vi "Update.vi"(8 "error in (no error)":errorcluster, 10 "TimePassed(ms)":i64, 11 "Timer in":refnum<class "Timer.lvclass">) -> (0 "error out":errorcluster, 1 "Triggered?":bool, 2 "UserEvent":T1, 3 "Timer out":refnum<class "Timer.lvclass">)   [LabVIEW 2017, in "TimerEngine.lvlib" / "Timer.lvclass"]
uses:
  Timer.lvclass
  _Typedef/Timer-UserEvent.ctl
  Timer.lvclass/Timer.ctl
  TimerEngine.lvclass
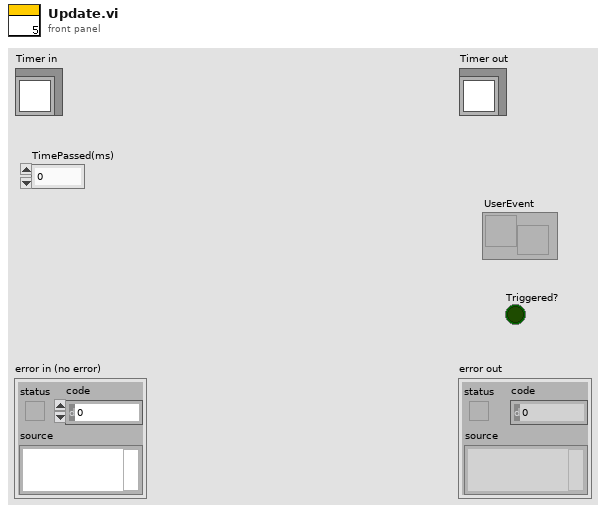
[diagram p1: front panel]
types:
  T1 = typedef "TimerEngine.lvlib/TimerEngine.lvclass/Timer-UserEvent.ctl" = refnum<user-event>
  T2 = typedef "TimerEngine.lvlib/TimerEngine.lvclass/Timer-Userevent.ctl" = refnum<user-event>
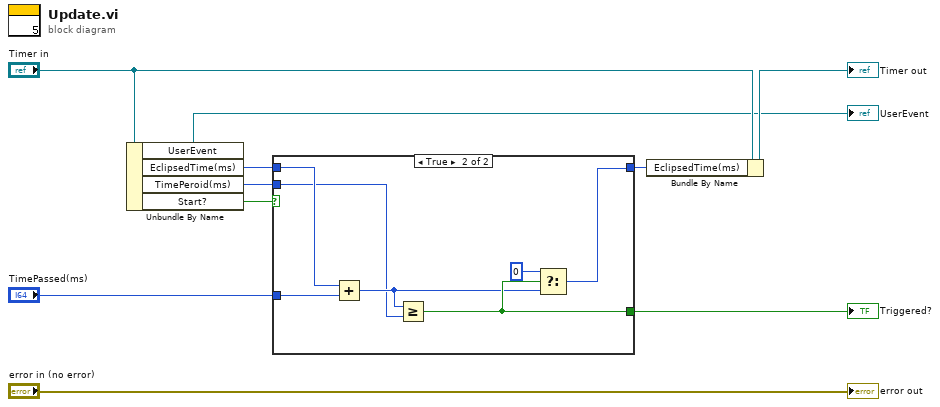
[diagram p0: block diagram]
diagram:
  n1 = Unbundle By Name("Timer in") -> ("UserEvent"=→"UserEvent":T2, "EclipsedTime(ms)"=w9:i64, "TimePeroid(ms)"=w7:i64, "Start?"=w1:bool)
  n2 = case shown="True" w1 {
    tunnel: w9 -> [_ w17]
    tunnel: [_ w16] -> w8
    tunnel: w7 -> [_ w14]
    tunnel: "TimePassed(ms)" -> [_ w13]
    tunnel: [_ w11] -> w5
    frame False {
    }
    frame True {
      n3 = Add(x=w17, y=w13) -> (x+y=w15:i64)
      n4 = Greater Or Equal?(x=w15, y=w14) -> (x >= y?=w16:bool)
      n5 = Select(t=i64 0, s=w16, f=w15) -> (s? t:f=w11:i64)
    }
  }
  "Triggered?" <- w8
  n6 = Bundle By Name(cluster="Timer in", "EclipsedTime(ms)"=w5) -> (→"Timer out":refnum<class "Timer.lvclass">)
  "error out" <- "error in (no error)"
